vi "Main.Create XNET Data Sessions.vi"(6 "Data":T1 {"IncomingDataRefs"."Data Reference" format="%.0x"; "OutgoingDataRefs"."Data Reference" format="%.0x"}, 8 "error in (no error)":errorcluster, 9 "Network":T5 {"Name" format="%.0x"}, 10 "J1939 XNET Settings":T6 {"Termination" items=["Off", "On"]}, 11 "DataTableLUT":variant) -> (0 "error out":errorcluster, 2 "XNET Sessions":T7 {"Network"."Name" format="%.0x"; "IncomingRefs"."Data Reference" format="%.0x"; "OutgoingRefs"."Data Reference" format="%.0x"}, 3 "DataTableLUT":variant)   [LabVIEW 2015, in "J1939 Addon Engine.lvlib"]
uses:
  J1939 Addon Engine.lvlib
  Types/Protocol.XNET Refs.ctl
  <vilib>/NI Veristand/Custom Device API/Block Data Reference.ctl
  <vilib>/NI Veristand/Custom Device API/Data Reference.ctl
  Shared/Types/Monitor Settings.ctl
  Shared/Types/XNET Settings.ctl
  Shared/Types/Device Settings.ctl
  Shared/Types/Frame Settings.ctl
  <vilib>/xnet/xnet.llb/XNET Control Scope.ctl
  <vilib>/xnet/xnet.llb/XNET Create Session (Signal Output Single-point).vi
  <vilib>/xnet/xnet.llb/XNET Create Session (Signal Input Single-point).vi
  <resource>/objmgr/xnet.rc
  <vilib>/NI VeriStand/Custom Device API/Custom Device API.lvlib
  Shared/J1939 Addon Shared.lvlib
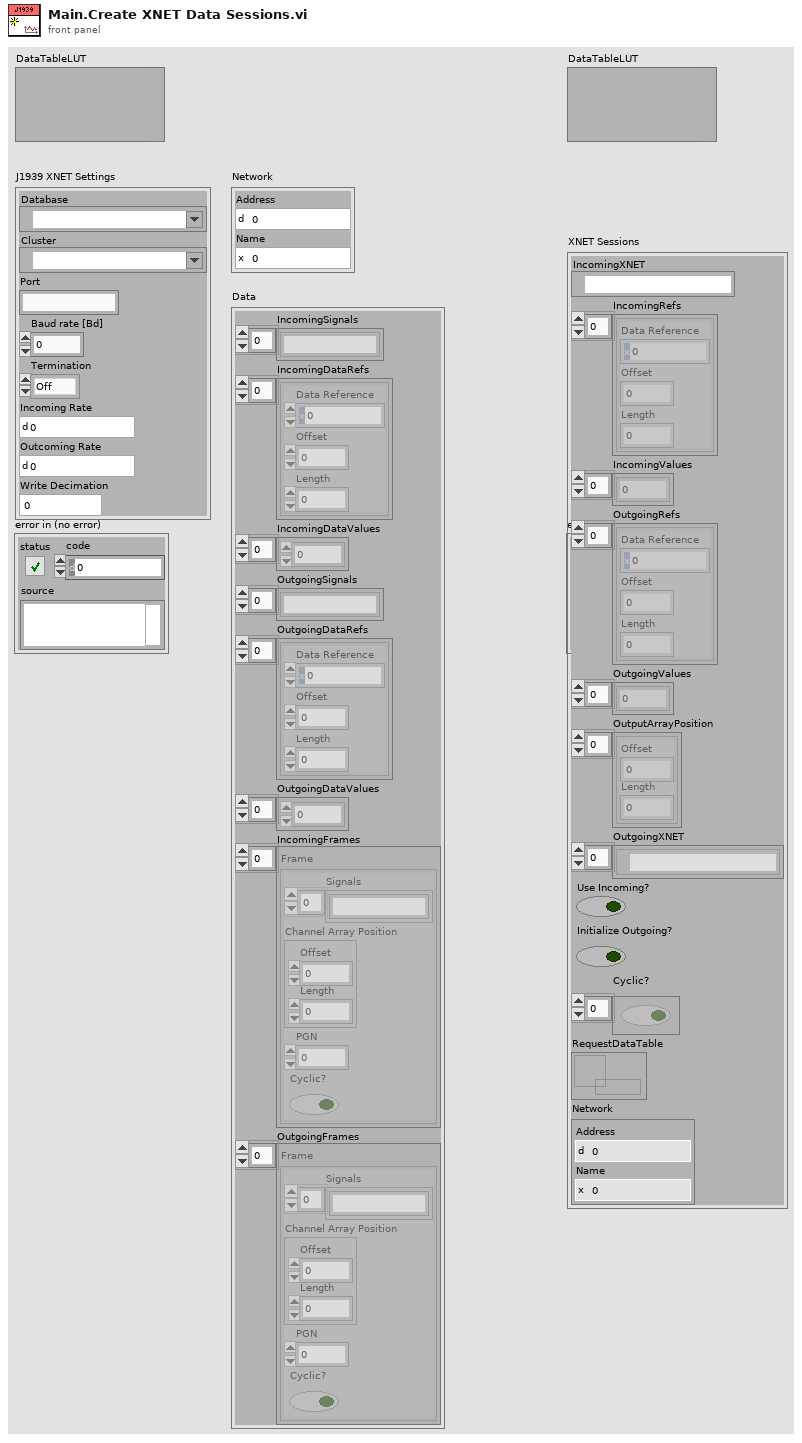
[diagram p1: front panel]
types:
  T1 = typedef "J1939 Addon Shared.lvlib/Device Settings.ctl" = cluster{"IncomingSignals":string[], "IncomingDataRefs":T2[], "IncomingDataValues":dbl[], "OutgoingSignals":string[], "OutgoingDataRefs":T2[], "OutgoingDataValues":dbl[], "IncomingFrames":T4[], "OutgoingFrames":T4[]}
  T2 = typedef "Custom Device API.lvlib/Block Data Reference.ctl" = cluster{"Data Reference":T3, "Offset":u64, "Length":u64}
  T3 = typedef "Custom Device API.lvlib/Data Reference.ctl" = i32
  T4 = typedef "J1939 Addon Shared.lvlib/Frame Settings.ctl" = cluster{"Signals":string[], "Channel Array Position":cluster{"Offset":u32, "Length":u32}, "PGN":u32, "Cyclic?":bool}
  T5 = typedef "J1939 Addon Shared.lvlib/Monitor Settings.ctl" = cluster{"Address":u8, "Name":u64}
  T6 = typedef "J1939 Addon Shared.lvlib/XNET Settings.ctl" = cluster{"Database":refnum<k21>, "Cluster":refnum<k21>, "Port":string, "Baud rate [Bd]":u32, "Termination":u32, "Incoming Rate":u32, "Outcoming Rate":u32, "Write Decimation":u32}
  T7 = typedef "J1939 Addon Engine.lvlib/Protocol.XNET Refs.ctl" = cluster{"IncomingXNET":refnum<k21>, "IncomingRefs":T2[], "IncomingValues":dbl[], "OutgoingRefs":T2[], "OutgoingValues":dbl[], "OutputArrayPosition":cluster{"Offset":u32, "Length":u32}[], "OutgoingXNET":refnum<k21>[], "Use Incoming?":bool, "Initialize Outgoing?":bool, "Cyclic?":bool[], "RequestDataTable":refnum<k33>, "Network":T5}
  T8 = cluster{"read mode":enum16{"polling", "blocking"}, "write mode":enum16{"polling", "blocking"}}
  T9 = typedef "XNET Control Scope.ctl" = u32
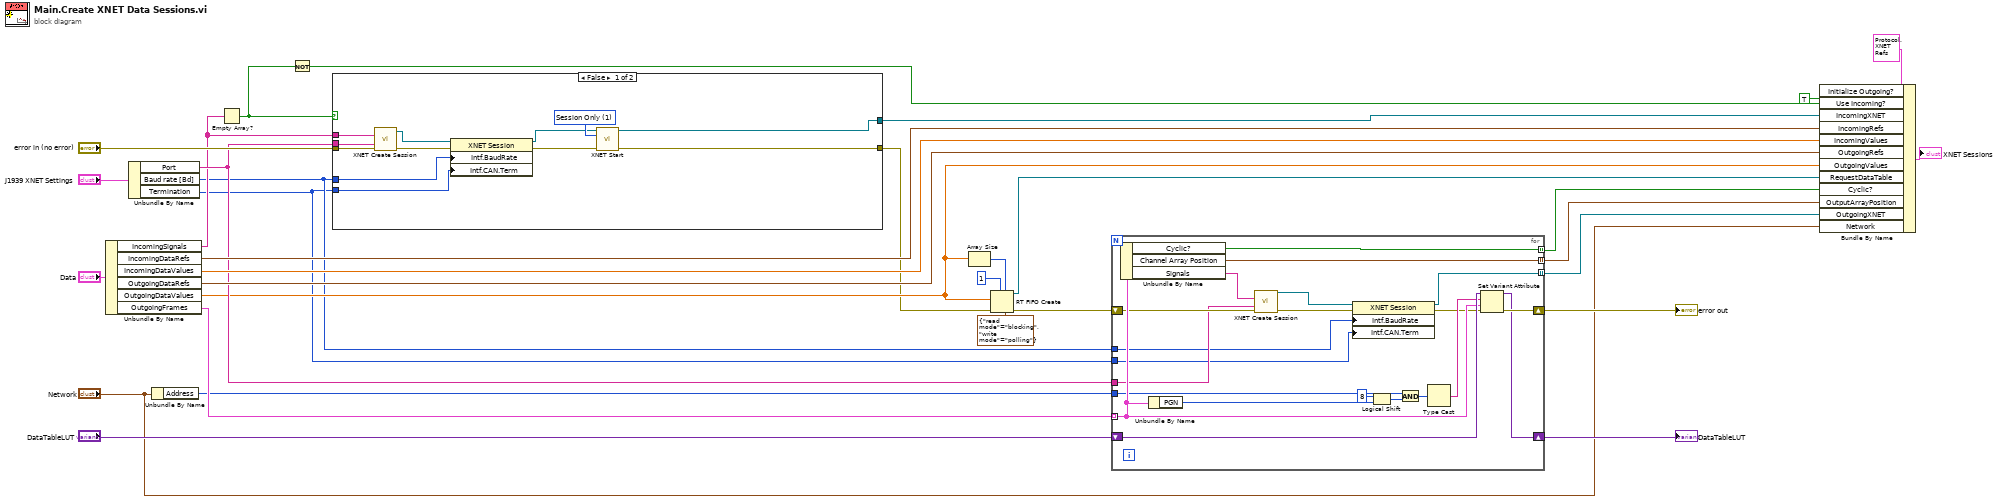
[diagram p0: block diagram]
diagram:
  n1 = Unbundle By Name("Data") -> ("IncomingSignals"=w18:string[], "IncomingDataRefs"=w24:T2[], "IncomingDataValues"=w23:dbl[], "OutgoingDataRefs"=w22:T2[], "OutgoingDataValues"=w12:dbl[], "OutgoingFrames"=w25:T4[])
  n2 = Unbundle By Name("J1939 XNET Settings") -> ("Port"=w19:string, "Baud rate [Bd]"=w5:u32, "Termination"=w4:u32)
  n3 = Unbundle By Name("Network") -> ("Address"=w21:u8)
  n4 = Empty Array?(array=w18) -> (empty?=w17:bool)
  n5 = Not(x=w17) -> (.not. x?=w16:bool)
  n6 = case shown="False" w17 {
    tunnel: [w33 _] -> w1
    tunnel: "error in (no error)" -> [w44 w45]
    tunnel: [w34 w45] -> w7
    tunnel: w19 -> [w43 _]
    tunnel: w18 -> [w42 _]
    tunnel: w5 -> [w37 _]
    tunnel: w4 -> [w36 _]
    frame False {
      w41 = T9 1 items=["Normal", "Session Only", "Interface Only", "Session Only Blocking"] ("scope (normal)")
      n7 = call-poly <vilib>:"XNET Create Session.vi"("signal list"=w42, "interface"=w43, "error in (no error)"=w44) -> ("session out"=w38:refnum<k21>, "error out"=w39:errorcluster)  [unwired: 11 in]
      n8 = property class="XNET Session"(reference=w38, error in=w39, "Intf.BaudRate"=w37, "Intf.CAN.Term"=w36) -> (reference out=w35:refnum<k21>, error out=w40:errorcluster)
      n9 = call <vilib>:"XNET Start.vi"("session in"=w35, "scope (normal)"=w41, "error in (no error)"=w40) -> ("session out"=w33:refnum<k21>, "error out"=w34:errorcluster)  [unwired: 11 in]
    }
    frame True {
    }
  }
  n10 = Array Size(array=w12) -> (size(s)=w11:i32)
  n11 = RT FIFO Create(1:w12, 3:w7, 4:1 ("max queue size (-1, unlimited)"), 6:w11, 7:T8 {"read mode"=enum."blocking", "write mode"=enum."polling"} ("r/w modes (polling,polling)")) -> (8:w8:refnum<k33>, 11:w13:errorcluster)  [unwired: 3 in, 1 out]
  n12 = for {
    tunnel: w25 -> [w58] mode=indexing
    tunnel: w21 -> [w53]
    shift-right: [w59] -> w32
    shift-left: "DataTableLUT" -> [w62]
    shift-right: [w60] -> w6
    shift-left: w13 -> [w56]
    tunnel: [w57] -> w20 mode=indexing
    tunnel: w19 -> [w55]
    tunnel: [w46] -> w2 mode=indexing
    tunnel: [w52] -> w14 mode=indexing
    tunnel: w5 -> [w49]
    tunnel: w4 -> [w48]
    n13 = Unbundle By Name(w58) -> ("Cyclic?"=w52:bool, "Channel Array Position"=w57:cluster{"Offset":u32, "Length":u32}, "Signals"=w54:string[])
    n14 = Unbundle By Name(w58) -> ("PGN"=w66:u32)
    n15 = call-poly <vilib>:"XNET Create Session.vi"("signal list"=w54, "interface"=w55, "error in (no error)"=w56) -> ("session out"=w50:refnum<k21>, "error out"=w51:errorcluster)  [unwired: 11 in]
    n16 = property class="XNET Session"(reference=w50, error in=w51, "Intf.BaudRate"=w49, "Intf.CAN.Term"=w48) -> (reference out=w46:refnum<k21>, error out=w47:errorcluster)
    n17 = Logical Shift(y=i16 8, x=w66) -> (x << y=w64:u32)
    n18 = And(x=w53, y=w64) -> (x .and. y?=w63:u32)
    n19 = Type Cast(x=w63) -> (*(type *) &x=w61:string)  [unwired: 1 in]
    n20 = Set Variant Attribute(Variant=w62, name=w61, value=w58, error in=w47) -> (Variant out=w59:variant, error out=w60:errorcluster)  [unwired: 1 out]
  }
  "error out" <- w6
  "DataTableLUT" <- w32
  n21 = Bundle By Name(cluster=T7 {"IncomingXNET"="", "IncomingRefs"=[], "IncomingValues"=[], "OutgoingRefs"=[], "OutgoingValues"=[], "OutputArrayPosition"=[], "OutgoingXNET"=[], "Use Incoming?"=FALSE, "Initialize Outgoing?"=FALSE, "Cyclic?"=[], "RequestDataTable"=refnum, "Network"={"Address"=0, "Name"=0}}, "Initialize Outgoing?"=TRUE, "Use Incoming?"=w16, "IncomingXNET"=w1, "IncomingRefs"=w24, "IncomingValues"=w23, "OutgoingRefs"=w22, "OutgoingValues"=w12, "RequestDataTable"=w8, "Cyclic?"=w14, "OutputArrayPosition"=w20, "OutgoingXNET"=w2, "Network"="Network") -> (→"XNET Sessions":T7)
